vi "Close ConvBox Handler.vi"(8 "error in (no error)":errorcluster, 11 "Listener in":refnum<class "Listener.lvclass">) -> (0 "error out":errorcluster, 3 "Listener out":refnum<class "Listener.lvclass">)   [LabVIEW 2019, in "Listener.lvclass"]
uses:
  Listener.lvclass
  Listener.lvclass/Listener.ctl
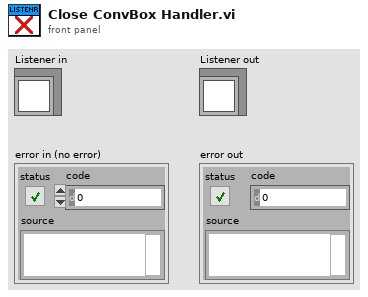
[diagram p1: front panel]
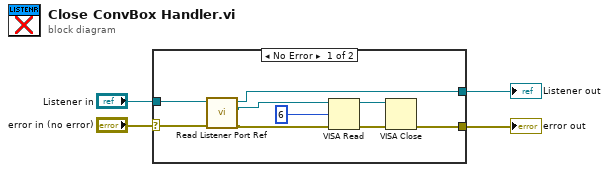
[diagram p0: block diagram]
diagram:
  n1 = case shown="No Error" "error in (no error)" {
    selector: "error in (no error)" -> [w8 w15]
    tunnel: [w12 w15] -> w3
    tunnel: "Listener in" -> [w9 w14]
    tunnel: [w5 w14] -> w1
    frame No Error {
      n2 = call "Read Listener Port Ref.vi"("error in (no error)"=w8, "Listener in"=w9) -> ("error out"=w7:errorcluster, "Listener Port Ref"=w6:refnum<visa-resource-name>, "Listener out"=w5:refnum<class "Listener.lvclass">)  [unwired: 7 in]
      n3 = VISA Read(VISA resource name=w6, byte count=u32 6, error in (no error)=w7) -> (VISA resource name out=w11:refnum<visa-resource-name>, error out=w10:errorcluster)  [unwired: 2 out]
      n4 = VISA Close(VISA resource name=w11, error in (no error)=w10) -> (error out=w12:errorcluster)
    }
    frame Error {
    }
  }
  "error out" <- w3
  "Listener out" <- w1
